vi "testSkip.vi"(8 "error in (no error)":errorcluster, 11 "TestCaseErrors":refnum<class "TestCaseErrors.lvclass">) -> (0 "error out":errorcluster, 3 "TestCaseErrors out":refnum<class "TestCaseErrors.lvclass">)   [LabVIEW 2013, in "TestCaseErrors.lvclass"]
uses:
  TestCaseErrors.lvclass
  Classes/TestCase/TestCase.lvclass
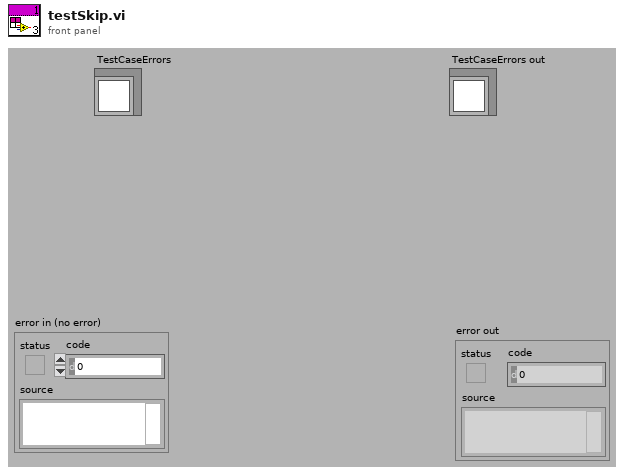
[diagram p1: front panel]
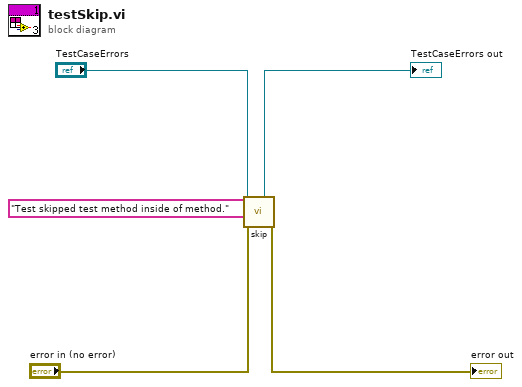
[diagram p0: block diagram]
diagram:
  n1 = call "skip.vi"("error in (no error)"="error in (no error)", "skipMessage"="Test skipped test method inside of method.", "TestCase in"="TestCaseErrors") -> ("error out"=→"error out":errorcluster, "TestCase out"=→"TestCaseErrors out":refnum<class "TestCaseErrors.lvclass">)  [unwired: 7 in]
